vi "VHDI-savingStatus.vi"(8 "error in (no error)":errorcluster, 10 "data saving info":T1={"data points left"=1, "Saving?"=FALSE, "Folder Path"=path "", "filename"=""}, 11 "VDHI-VNA_data_handler_interface in":refnum<class "VDHI-VNA_data_handler_interface.lvclass">) -> (0 "error out":errorcluster, 3 "VDHI-VNA_data_handler_interface out":refnum<class "VDHI-VNA_data_handler_interface.lvclass">)   [LabVIEW 2020, in "VDHI-VNA_data_handler_interface.lvlib" / "VDHI-VNA_data_handler_interface.lvclass"]
uses:
  VDHI-VNA_data_handler_interface.lvclass
  VDH-VNA_data_handler/VDH-VNA_data_handler/VDH-data_saving_info.ctl
  VDH-VNA_data_handler/VDH-VNA_data_handler/VDH-VNA_data_handler.lvclass
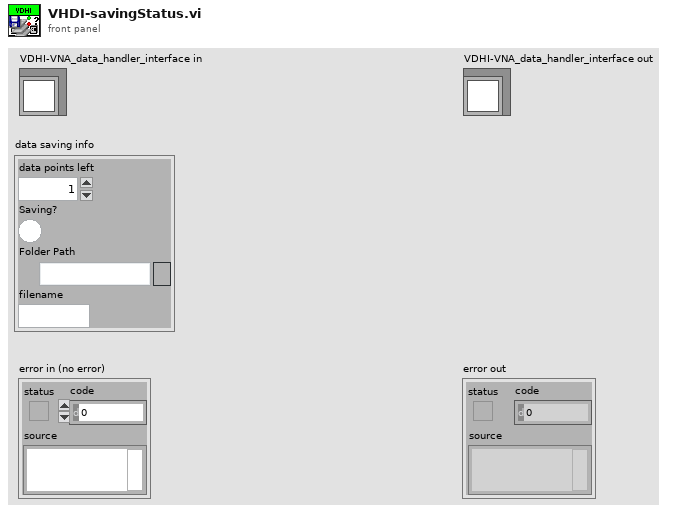
[diagram p1: front panel]
types:
  T1 = typedef "VDH-VNA_data_handler.lvlib/VDH-VNA_data_handler.lvclass/VDH-data_saving_info.ctl" = cluster{"data points left":u8, "Saving?":bool, "Folder Path":path, "filename":string}
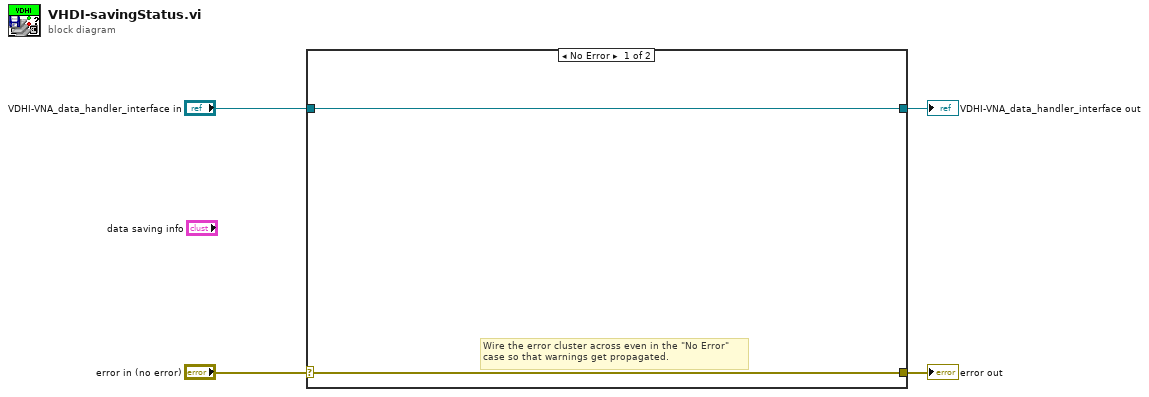
[diagram p0: block diagram]
diagram:
  n1 = case shown="No Error" "error in (no error)" {
    selector: "error in (no error)" -> [w5 w8]
    tunnel: [w5 w8] -> w3
    tunnel: [w6 w7] -> w1
    tunnel: "VDHI-VNA_data_handler_interface in" -> [w6 w7]
    frame No Error {
      # "Wire the error cluster across even in the \"No Error\"\ncase so that warnings get propagated."
    }
    frame Error {
    }
  }
  "error out" <- w3
  "VDHI-VNA_data_handler_interface out" <- w1
